vi "Read Test Report.vi"(11 "Test Manager in":refnum<class "Test Manager.lvclass">) -> (2 "Test Report":refnum<class "Test Report.lvclass">, 3 "Test Manager out":refnum<class "Test Manager.lvclass">)   [LabVIEW 2009, in "Caraya.lvlib" / "Test Manager.lvclass"]
uses:
  Test Manager.lvclass
  Test Report/Test Report.lvclass
  Test Manager.lvclass/Test Manager.ctl
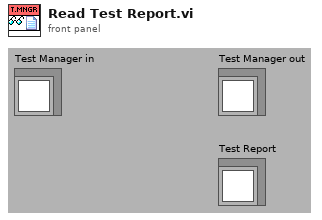
[diagram p1: front panel]
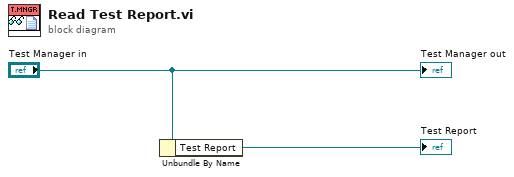
[diagram p0: block diagram]
diagram:
  n1 = Unbundle By Name("Test Manager in") -> ("Test Report"=→"Test Report":refnum<class "Test Report.lvclass">)
  "Test Manager out" <- "Test Manager in"
